vi "UDCLogUsageData.vi"(5 "LogMessageSize":T1, 7 "LogMessageFrequency":T2, 8 "Error In":errorcluster, 9 "KeyUID":string, 10 "Value":string, 11 "Key":string) -> (0 "Error Out":errorcluster)   [LabVIEW 2020, in "niceiplib.lvlib"]
doc: "This is the API that will log the CEIP messages in Key Value pairs. This API can log only when CEIP is already initialized. \n\nThere are two additional parameters that needs to be given.\n\nLogMessageFrequency :\nOncePerSession: Usually happens once per session\nLowFrequency: Low frequency events. Usually happens 2-5 times per session\nMediumFrequency: Happens more frequently per session. Usually 5-25 times per session\nHighFrequency: Highly frequently. 25-100 times per session\nKBMouseEvents: Polling actions. >100 log messages per session\n\nLogMessageSize\nSmallMessage: Small Log Messages < 50 characters in the value field\nMediumMessage: Medium Log Messages 50 - 300 characters in the value field\nLargeMessage: Large log messages > 300 characters in the value field. The limit is 1000 characters"
uses:
  <vilib>/UDC/niceiplib.lvlib
  <vilib>/UDC/Controls/LogMessageFrequency.ctl
  <vilib>/UDC/Controls/LogMessageSize.ctl
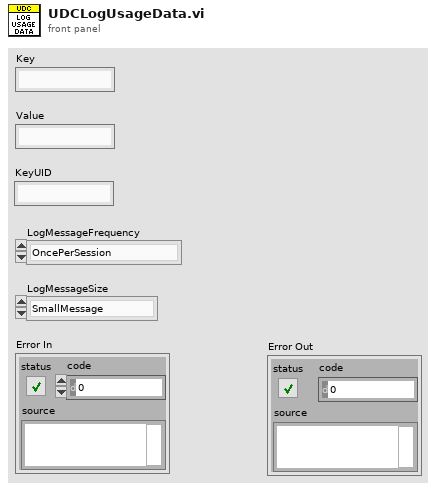
[diagram p1: front panel]
types:
  T1 = typedef "niceiplib.lvlib/LogMessageSize.ctl" = enum32{"SmallMessage", "MediumMessage", "LargeMessage"}
  T2 = typedef "niceiplib.lvlib/LogMessageFrequency.ctl" = enum32{"OncePerSession", "LowFrequency", "MediumFrequency", "HighFrequency", "KBMouseEvents"}
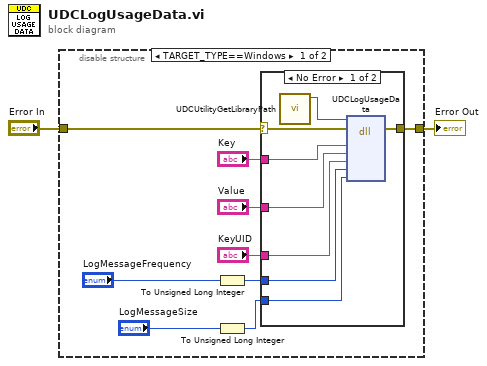
[diagram p0: block diagram]
diagram:
  n1 = disable-structure shown="TARGET_TYPE==Windows" {
    disable-tunnel: [w5 w21] -> w2
    disable-tunnel: "Error In" -> [w4 w21]
    frame condition #0 (active) {
      n2 = To Unsigned Long Integer(number="LogMessageFrequency") -> (unsigned 32bit integer=w7:u32)
      n3 = To Unsigned Long Integer(number="LogMessageSize") -> (unsigned 32bit integer=w6:u32)
      n4 = case shown="No Error" w4 {
        selector: w4 -> [w14 w20]
        tunnel: "Key" -> [w19 _]
        tunnel: "Value" -> [w18 _]
        tunnel: w7 -> [w17 _]
        tunnel: w6 -> [w16 _]
        tunnel: [w15 w20] -> w5
        tunnel: "KeyUID" -> [w12 _]
        frame No Error {
          n5 = call <vilib>:"UDCUtilityGetLibraryPath.vi"() -> ("Library Path"=w13:path)  [unwired: 11 in]
          n6 = dll-call lib="C:/2013LabVIEWCode/dist/vi.lib/UDC/niceiplib.dll" fn="UDCLogUsageData"(path in=w13, error in=w14, "Key"=w19, "Value"=w18, "KeyUID"=w12, "MessageFrequency"=w17, "MessageSize"=w16) -> (error out=w15:errorcluster)  [unwired: 7 in, 1 out]
        }
        frame Error {
        }
      }
    }
    frame condition #1 {
    }
  }
  "Error Out" <- w2
